vi "Read Connection Ref.vi"(8 "error in (no error)":errorcluster, 11 "PXI 8513 in":refnum<class "PXI 8513.lvclass">) -> (0 "error out":errorcluster, 2 "Connection Ref":variant, 3 "PXI 8513 out":refnum<class "PXI 8513.lvclass">)   [LabVIEW 2021, in "CAN.lvlib" / "PXI 8513.lvclass"]
uses:
  PXI 8513.lvclass
  PXI 8513.lvclass/PXI 8513.ctl
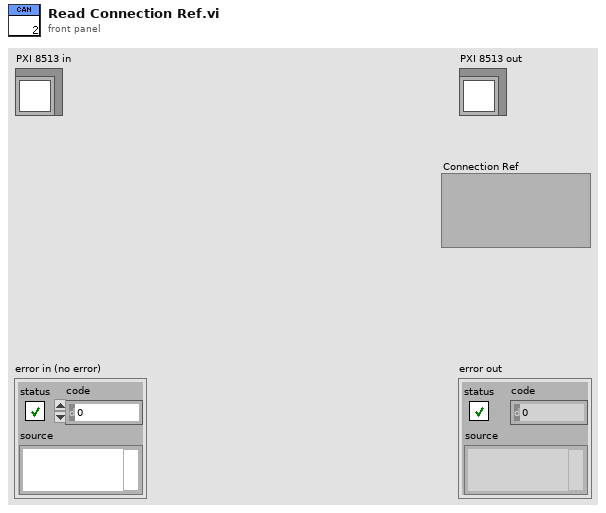
[diagram p1: front panel]
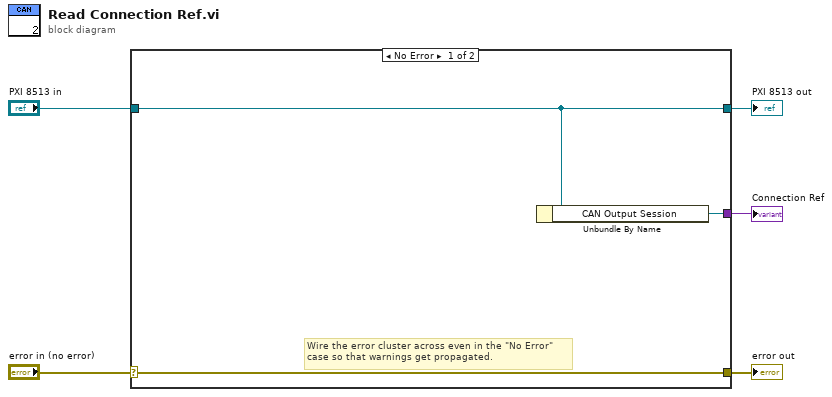
[diagram p0: block diagram]
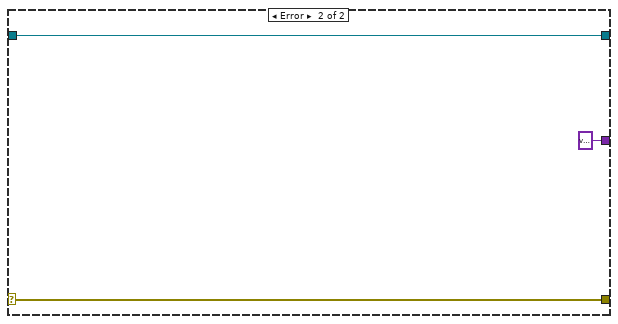
[diagram p2: hidden frame]
diagram:
  n1 = case shown="No Error" "error in (no error)" {
    selector: "error in (no error)" -> [w8 w11]
    tunnel: [w8 w11] -> w4
    tunnel: [w7 w10] -> w2
    tunnel: "PXI 8513 in" -> [w7 w10]
    tunnel: [w6 variant ("Connection Ref")] -> w1
    frame No Error {
      # "Wire the error cluster across even in the \"No Error\"\ncase so that warnings get propagated."
      n2 = Unbundle By Name(w7) -> ("CAN Output Session"=w6:refnum<k21>)
    }
    frame Error {
    }
  }
  "error out" <- w4
  "PXI 8513 out" <- w2
  "Connection Ref" <- w1
